vi "Set Pause.vi"(8 "error in (no error)":errorcluster, 10 "Pause":bool, 11 "FormulaG API in":refnum<class "FormulaG API.lvclass">) -> (0 "error out":errorcluster, 3 "FormulaG API out":refnum<class "FormulaG API.lvclass">)   [LabVIEW 2020, in "FormulaG.lvlib" / "FormulaG API.lvclass"]
uses:
  FormulaG API.lvclass
  Command.ctl
  FormulaG API.lvclass/FormulaG API.ctl
  <vilib>/IlluminatedG/lv-stream/stream/Stream.lvclass/Stream.ctl
  <vilib>/IlluminatedG/lv-stream/stream/Dispatch Sniffer Data.vi
  <vilib>/IlluminatedG/lv-stream/stream/Prepared.vi
  <vilib>/IlluminatedG/lv-stream/Endpoint/Cast Sniffer Callback.vi
  <vilib>/IlluminatedG/IG WebSocket Stream/Stream-Websocket/WebsocketStream/WebsocketStream.lvclass
  C:/Program Files (x86)/National Instruments/LabVIEW 2020/vi.lib/IlluminatedG/lv-stream/stream/Stream.lvclass
  <vilib>/Utility/error.llb/Error Cluster From Error Code.vi
  <vilib>/IlluminatedG/lv-stream/stream/Stream.lvclass
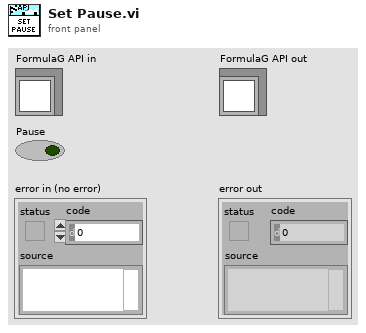
[diagram p1: front panel]
types:
  T1 = enum16{"big-endian, network order", "native, host order", "little-endian"}
  T2 = typedef "FormulaG.lvlib/FormulaG API.lvclass/Command.ctl" = enum8{"None", "Reset Car", "Request Ranges", "Control Car", "Request Info", "Set Options", "Set Camera", "Set Pause", "Request Time"}
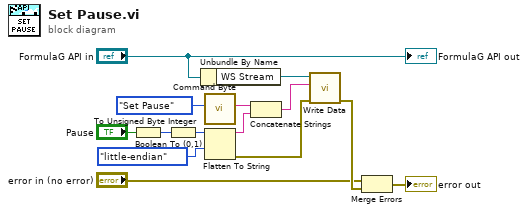
[diagram p0: block diagram]
diagram:
  n1 = Boolean To (0,1)(Boolean="Pause") -> (0, 1=w5:i16)
  n2 = To Unsigned Byte Integer(number=w5) -> (unsigned 8bit integer=w4:u8)
  n3 = Unbundle By Name("FormulaG API in") -> ("WS Stream"=w12:refnum<class "WebsocketStream.lvclass">)
  n4 = call "Command Byte.vi"("Command"=Command."Set Pause") -> ("Command Byte"=w13:string)  [unwired: 10 in]
  n5 = Flatten To String(anything=w4, byte order (0:big-endian, network order)=T1."little-endian") -> (data string=w9:string, error out=w8:errorcluster)  [unwired: 2 in, 1 out]
  n6 = Concatenate Strings(w13, w9) -> (w11:string)
  n7 = call <vilib>:"Write Data.vi"("error in (no error)"=w8, "Data"=w11, "Stream in"=w12) -> ("error out"=w7:errorcluster)  [unwired: 7 in, 1 out]
  n8 = Merge Errors("error in (no error)", w7) -> (→"error out":errorcluster)
  "FormulaG API out" <- "FormulaG API in"
